vi "ChipKit Seven Segment Display.vi"() -> ()   [LabVIEW 2011, in "LabVIEW Interface for ChipKit.lvlib"]
doc: "This example demonstrates how to use the digital output pins of the ChipKit to control a seven segment display."
uses:
  vi.lib/LabVIEW Interface for ChipKit/LabVIEW Interface for ChipKit.lvlib
  vi.lib/LabVIEW Interface for ChipKit/Private/Type Defs/Chipkit Configuration.ctl
  vi.lib/LabVIEW Interface for ChipKit/Private/Type Defs/Board Type.ctl
panel:
  in  "ChipKit Configuration":T1
  in  "Delay between Characters (ms)":u32=500
  in  "Message":string="Hello"
  in  "Stop Button":bool
  # "chipKIT Settings"
  # "Seven Segment LED Settings"
  # "7-Segment Display Example\n\nThis example demonstrates how to write scrolling text to a seven segment display.\n\nInstructions\n1. Select the COM Port associated with the ChipKit.\n2. Select the Board Type.\n3. Click the Run Arrow.\n4. Change the Message to write different text (Note: Not all characters are possible on the display)\n5. Change the Delay to adjust the 'scroll speed'."
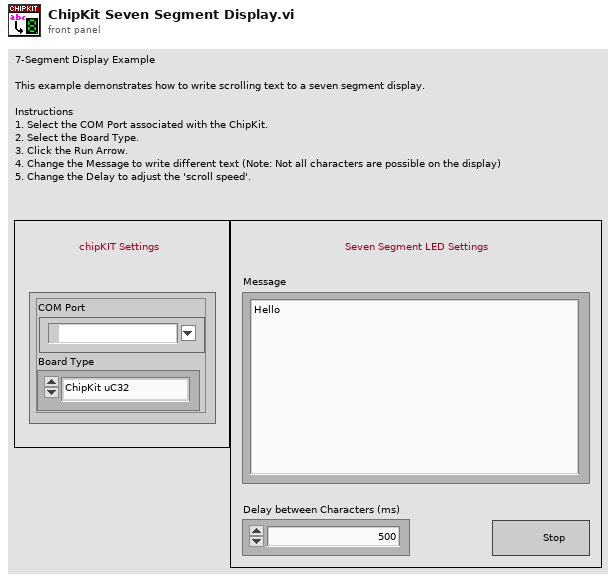
[diagram p1: front panel]
types:
  T1 = typedef "LabVIEW Interface for ChipKit.lvlib/Chipkit Configuration.ctl" = cluster{"COM Port":refnum<visa-resource-name>, "Board Type":T2}
  T2 = typedef "LabVIEW Interface for ChipKit.lvlib/Board Type.ctl" = enum16{"ChipKit uC32", "ChipKit Uno32", "ChipKit Max32"}
  T3 = typedef "LabVIEW Interface for ChipKit.lvlib/Chipkit Resource.ctl" = cluster{"COM Port":refnum<visa-resource-name>, "Board Type":T2, "Connection Type":T4, "Baud Rate (115200)":u32, "Bytes Per Packet (15)":u32, "DI Port Num Pins":i32, "DO Port Num Pins":i32}
  T4 = typedef "LabVIEW Interface for ChipKit.lvlib/Connection Type.ctl" = enum8{"USB / Serial", "XBEE", "BlueSmirf (Bluetooth)"}
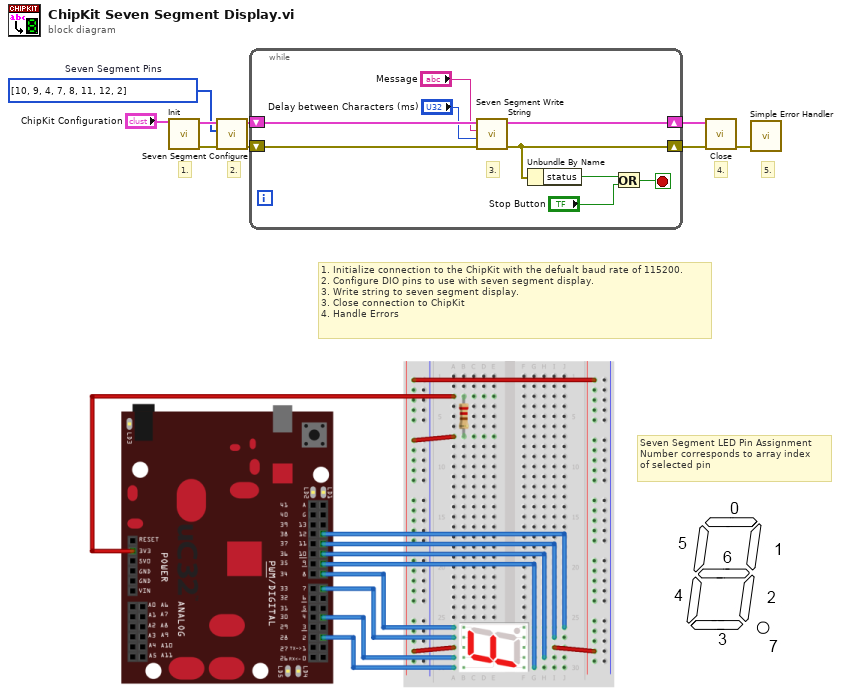
[diagram p0: block diagram]
diagram:
  w2 = u8[] [10, 9, 4, 7, 8, 11, 12, 2]  # Seven Segment Pins
  # "Seven Segment LED Pin Assignment\nNumber corresponds to array index\nof selected pin"
  # "5."
  # "4."
  # "2."
  # "1."
  # "1. Initialize connection to the ChipKit with the defualt baud rate of 115200.\n2. Configure DIO pins to use with seven segment display. \n3. Write string to seven segment display.\n3. Close connection to ChipKit\n4. Handle Errors"
  n1 = call "Init.vi"("ChipKit Configuration"="ChipKit Configuration") -> ("Error Out"=w6:errorcluster, "ChipKit Configuration"=w3:T3)  [unwired: 9 in]
  n2 = call "Seven Segment Configure.vi"("Error In"=w6, "Seven Segment Pins"=w2, "ChipKit Resource"=w3) -> ("Error Out"=w7:errorcluster, "ChipKit Resource"=w8:T3)  [unwired: 7 in]
  n3 = while {
    shift-right: [w18] -> w4
    shift-left: w8 -> [w14]
    shift-right: [w10] -> w9
    shift-left: w7 -> [w17]
    stop <- w16 stop-if-true
    # "3."
    n4 = call "Seven Segment Write String.vi"("Error In"=w17, "Delay (500)"="Delay between Characters (ms)", "Message"="Message", "ChipKit Resource"=w14) -> ("Error Out"=w10:errorcluster, "ChipKit Resource"=w18:T3)  [unwired: 6 in]
    n5 = Unbundle By Name(w10) -> ("status"=w15:bool)
    n6 = Or(x=w15, y="Stop Button") -> (x .or. y?=w16:bool)
  }
  n7 = call "Close.vi"("Error In"=w9, "ChipKit Configuration"=w4) -> ("Error Out"=w5:errorcluster)  [unwired: 9 in]
  n8 = call <vilib>:"Simple Error Handler.vi"("error in (no error)"=w5) -> ()  [unwired: 4 in, 5 out]
